vi "Layer1d.vi"(7 "Activation Function":enum32{"Sigmoid", "RELU", "Tanh", "Leaky RELU"}(radio), 9 "Biases":dbl, 10 "Weights":dbl[](array[numeric]), 11 "Data":dbl[](array[numeric])) -> (0 "Error":i32, 2 "Net Activation":dbl, 3 "Output":dbl)   [LabVIEW 2019]
uses:
  Globals.vi
  <vilib>/Analysis/NI_AALBase.lvlib
  <vilib>/Analysis/baseanly.llb/Real Dot Product.vi
panel:
  out "size(s) 2":i32
  out "size(s)":i32
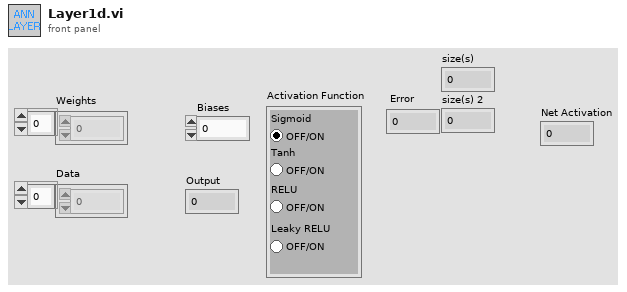
[diagram p1: front panel]
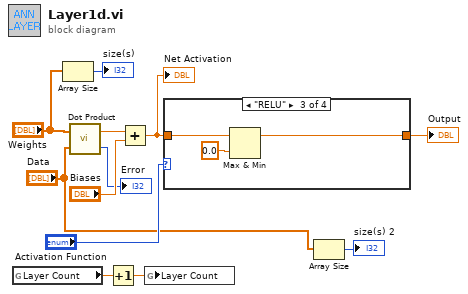
[diagram p0: block diagram]
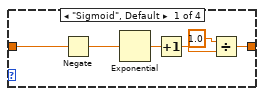
[diagram p2: hidden frame]
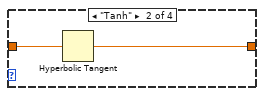
[diagram p3: hidden frame]
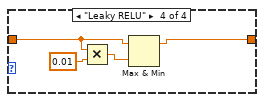
[diagram p4: hidden frame]
diagram:
  n1 = global read "Globals.vi" "Layer Count"() -> (w10:dbl)
  n2 = Array Size(array="Weights") -> (size(s)=→"size(s)":i32)
  n3 = call-poly <vilib>:"Dot Product.vi"("Y Vector"="Data", "X Vector"="Weights") -> ("error"=→"Error":i32, "X * Y"=w8:dbl)
  n4 = Increment(x=w10) -> (x+1=w9:dbl)
  n5 = Add(x=w8, y="Biases") -> (x+y=w6:dbl)
  "Net Activation" <- w6
  n6 = global write "Globals.vi" "Layer Count"(w9) -> ()
  n7 = case shown="\"RELU\"" "Activation Function" {
    tunnel: [w14 w20 w21 w24] -> w7
    tunnel: w6 -> [w13 w19 w22 w25]
    frame "Sigmoid", Default {
      n8 = Negate(x=w13) -> (-x=w16:dbl)
      n9 = Exponential(1:w16) -> (0:w15:dbl)
      n10 = Increment(x=w15) -> (x+1=w17:dbl)
      n11 = Divide(x=1.0, y=w17) -> (x/y=w14:dbl)
    }
    frame "Tanh" {
      n12 = Hyperbolic Tangent(1:w19) -> (0:w20:dbl)
    }
    frame "RELU" {
      n13 = Max & Min(x=w22, y=0.0) -> (max(x,y)=w21:dbl)  [unwired: 1 out]
    }
    frame "Leaky RELU" {
      n14 = Multiply(x=w25, y=0.01) -> (x*y=w26:dbl)
      n15 = Max & Min(x=w25, y=w26) -> (max(x,y)=w24:dbl)  [unwired: 1 out]
    }
  }
  "Output" <- w7
  n16 = Array Size(array="Data") -> (size(s)=→"size(s) 2":i32)
